vi "cam0-从起始钩角计算所有槽角.vi"(7 "中心点":cluster{"X":i32, "Y":i32}, 9 "钩子起始角度":dbl format="%#_13g", 10 "槽数":i32=3, 11 "ImageIN":T1) -> (2 "各槽角":dbl[](array[numeric]), 3 "ImageOUT":T1)   [LabVIEW 2018]
uses:
  <vilib>/vision/Image Controls.llb/IMAQ Image.ctl
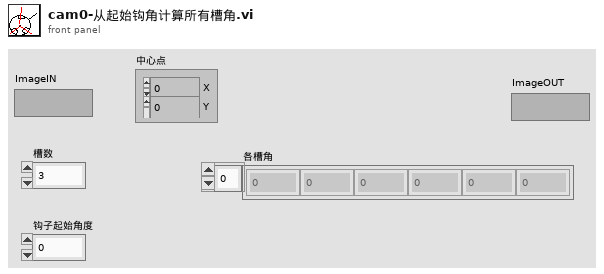
[diagram p1: front panel]
types:
  T1 = typedef "IMAQ Image.ctl" = refnum<image>
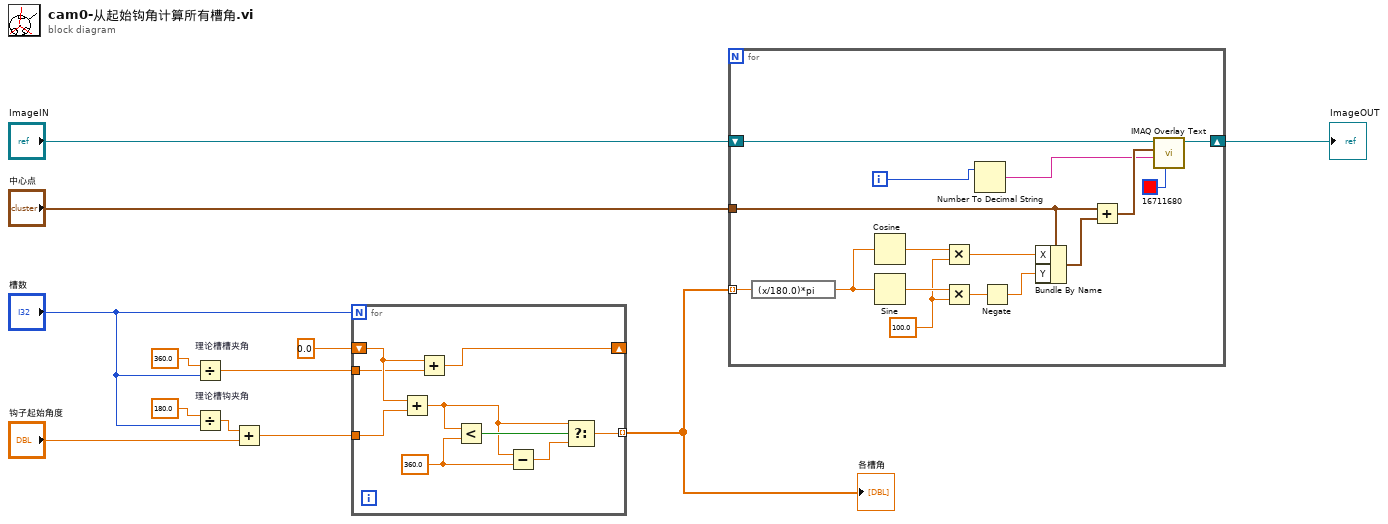
[diagram p0: block diagram]
diagram:
  n1 = Divide "理论槽槽夹角"(x=360.0, y="槽数") -> (x/y=w6:dbl)
  n2 = Divide "理论槽钩夹角"(x=180.0, y="槽数") -> (x/y=w11:dbl)
  n3 = Add(x=w11, y="钩子起始角度") -> (x+y=w9:dbl)
  n4 = for {
    N: "槽数" -> [_]
    tunnel: w6 -> [w14]
    tunnel: w9 -> [w21]
    tunnel: [w16] -> w4 mode=indexing
    shift-right: [w13] -> _
    shift-left: 0.0 -> [w15]
    w18 = 360.0 ("x")
    n5 = Add(x=w15, y=w21) -> (x+y=w19:dbl)
    n6 = Add(x=w15, y=w14) -> (x+y=w13:dbl)
    n7 = Less?(x=w19, y=w18) -> (x < y?=w20:bool)
    n8 = Subtract(x=w19, y=w18) -> (x-y=w17:dbl)
    n9 = Select(t=w19, s=w20, f=w17) -> (s? t:f=w16:dbl)
  }
  "各槽角" <- w4
  n10 = for {
    tunnel: w4 -> [w25] mode=indexing
    shift-right: [w36] -> w2
    shift-left: "ImageIN" -> [w37]
    tunnel: "中心点" -> [w30]
    i -> [w28]
    w33 = 100.0 ("y")
    n11 = expression code="(x/180.0)*pi" ("degrees to radians")(w25) -> (w24:dbl)
    n12 = Cosine(x=w24) -> (cos(x)=w34:dbl)
    n13 = Sine(x=w24) -> (sin(x)=w35:dbl)
    n14 = Multiply(x=w34, y=w33) -> (x*y=w32:dbl)
    n15 = Multiply(x=w35, y=w33) -> (x*y=w23:dbl)
    n16 = Number To Decimal String(number=w28) -> (decimal integer string=w27:string)  [unwired: 1 in]
    n17 = Negate(x=w23) -> (-x=w22:dbl)
    n18 = Bundle By Name(cluster=w30, "X"=w32, "Y"=w22) -> (w31:cluster{"X":i32, "Y":i32})
    n19 = Add(x=w30, y=w31) -> (x+y=w29:cluster{"X":i32, "Y":i32})
    n20 = call "IMAQ Overlay Text"("Text Color (black)"=u32 16711680, "String"=w27, "Origin"=w29, "Image"=w37) -> ("Image Out"=w36:T1)  [unwired: 6 in, 1 out]
  }
  "ImageOUT" <- w2
